vi "global_stop.vi"() -> ()   [LabVIEW 2017]
panel:
  out "Stop Boolean":bool
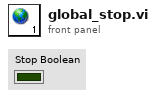
[diagram p1: front panel]
diagram:
